vi "AlliGator Get tau1, tau2 & a1.vi"(10 "Best Fit Parameters":dbl[](array[numeric])) -> (0 "a 1":dbl, 1 "tau 2":dbl, 2 "tau 1":dbl)   [LabVIEW 2021, in "AlliGator Fit Method Benchmark.lvlib"]
doc: "Outputs tau1, tau2 and a1."
uses:
  AlliGator Fit Method Benchmark.lvlib
panel:
  # "see the AlliGator License on the block diagram (Ctrl+E or Window:Show Block Diagram)"
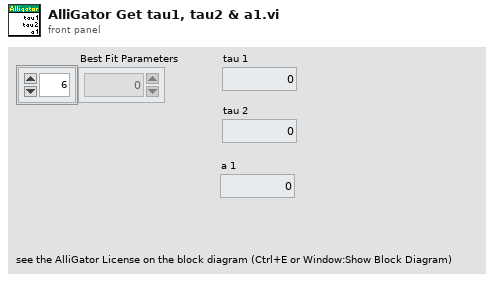
[diagram p1: front panel]
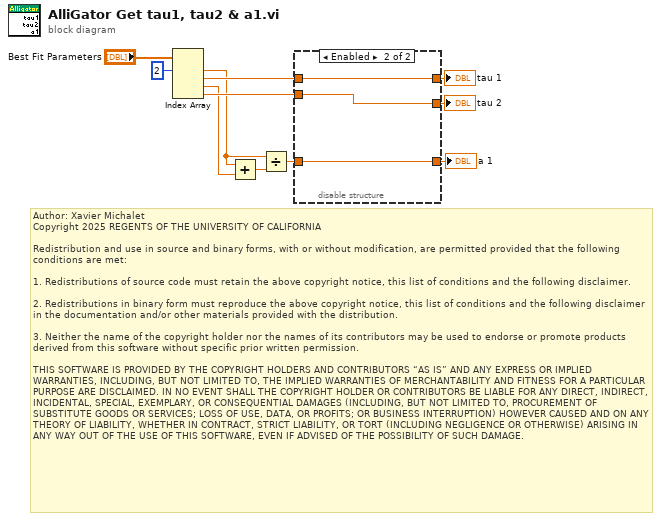
[diagram p0: block diagram]
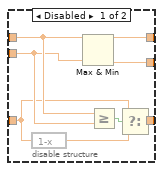
[diagram p2: hidden frame]
diagram:
  # "Author: Xavier Michalet\nCopyright 2025 REGENTS OF THE UNIVERSITY OF CALIFORNIA\n\nRedistribution and use in source and binary forms, with or without modification, are permitted provided that the following conditions are met:\n\n1. Redistributions of source code must retain the above copyright notice, this list of conditions and the following disclaimer.\n\n2. Redistributions in binary form must reproduce the above copyright notice, this list of conditions and the following disclaimer in the documentation and/or other materials provided with the distribution.\n\n3. Neither the name of the copyright holder nor the names of its contributors may be used to endorse or promote products derived from this software without specific prior written permission.\n\nTHIS SOFTWARE IS PROVIDED BY THE COPYRIGHT HOLDERS AND CONTRIBUTORS “AS IS” AND ANY EXPRESS OR IMPLIED WARRANTIES, INCLUDING, BUT NOT LIMITED TO, THE IMPLIED WARRANTIES OF MERCHANTABILITY AND FITNESS FOR A PARTICULAR PURPOSE ARE DISCLAIMED. IN NO EVENT SHALL THE COPYRIGHT HOLDER OR CONTRIBUTORS BE LIABLE FOR ANY DIRECT, INDIRECT, INCIDENTAL, SPECIAL, EXEMPLARY, OR CONSEQUENTIAL DAMAGES (INCLUDING, BUT NOT LIMITED TO, PROCUREMENT OF SUBSTITUTE GOODS OR SERVICES; LOSS OF USE, DATA, OR PROFITS; OR BUSINESS INTERRUPTION) HOWEVER CAUSED AND ON ANY THEORY OF LIABILITY, WHETHER IN CONTRACT, STRICT LIABILITY, OR TORT (INCLUDING NEGLIGENCE OR OTHERWISE) ARISING IN ANY WAY OUT OF THE USE OF THIS SOFTWARE, EVEN IF ADVISED OF THE POSSIBILITY OF SUCH DAMAGE."
  n1 = Index Array(array="Best Fit Parameters", index #1=2 ("index")) -> (element #1=w1:dbl, element #2=w7:dbl, element #3=w4:dbl, element #4=w6:dbl)  [unwired: 3 in]
  n2 = Add(x=w1, y=w4) -> (x+y=w3:dbl)
  n3 = Divide(x=w1, y=w3) -> (x/y=w2:dbl)
  n4 = disable-structure shown="Enabled" {
    disable-tunnel: [w19 w21] -> w11
    disable-tunnel: [w18 w22] -> w10
    disable-tunnel: w7 -> [w17 w22]
    disable-tunnel: w6 -> [w16 w21]
    disable-tunnel: [w15 w20] -> w5
    disable-tunnel: w2 -> [w14 w20]
    frame Disabled {
      n5 = expression code="1-x"(w14) -> (w12:dbl)
      n6 = Max & Min(x=w17, y=w16) -> (max(x,y)=w18:dbl, min(x,y)=w19:dbl)
      n7 = Greater Or Equal?(x=w17, y=w16) -> (x >= y?=w13:bool)
      n8 = Select(t=w14, s=w13, f=w12) -> (s? t:f=w15:dbl)
    }
    frame Enabled {
    }
  }
  "a 1" <- w5
  "tau 2" <- w11
  "tau 1" <- w10
